vi "Filter Path Node.vi"(7 "Node Path Type":string="To Common Doc Dir", 8 "error in":errorcluster, 11 "Nodes Array in":refnum<k20>[](array[refnum])) -> (0 "error out":errorcluster, 3 "Nodes Array out":refnum<k20>[](array[refnum]))   [LabVIEW 2018, in ".LVLIBP CD XML Updater.lvlib" / "Project XML Editor.lvclass"]
uses:
  Project XML Editor.lvclass
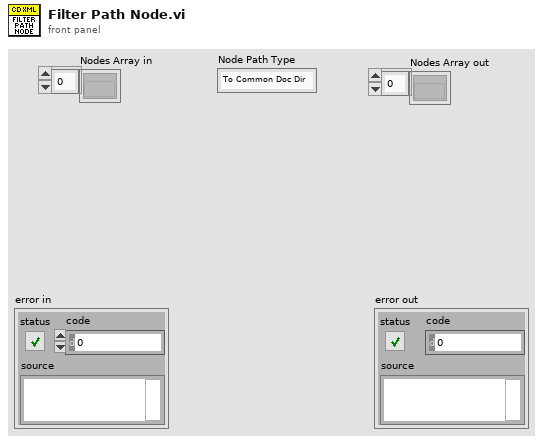
[diagram p1: front panel]
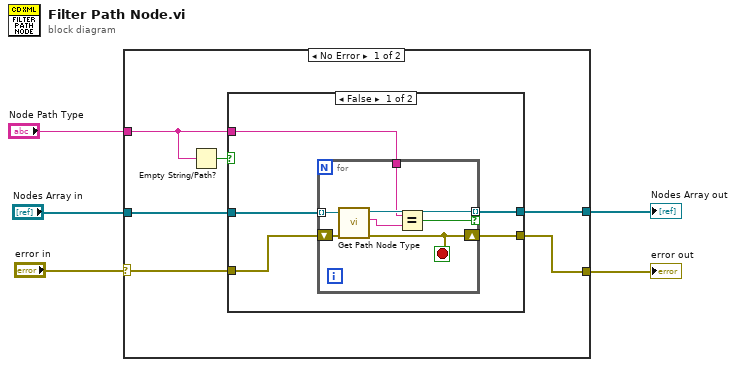
[diagram p0: block diagram]
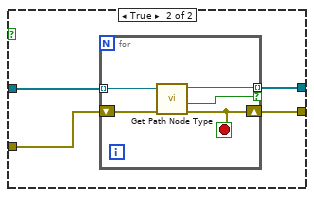
[diagram p2: hidden frame]
diagram:
  n1 = case shown="No Error" "error in" {
    selector: "error in" -> [w8 w33]
    tunnel: "Nodes Array in" -> [w11 w34]
    tunnel: [w10 w34] -> w4
    tunnel: [w9 w33] -> w3
    tunnel: "Node Path Type" -> [w7 _]
    frame No Error {
      n2 = Empty String/Path?(string/path=w7) -> (empty?=w6:bool)
      n3 = case shown="False" w6 {
        tunnel: w11 -> [w16 w27]
        tunnel: [w15 w25] -> w10
        tunnel: [w14 w24] -> w9
        tunnel: w8 -> [w13 w26]
        tunnel: w7 -> [w12 _]
        frame False {
          n4 = for {
            tunnel: [w23] -> w15 mode=indexing if=w22
            tunnel: w16 -> [w21] mode=indexing
            shift-right: [w18] -> w14
            shift-left: w13 -> [w20]
            tunnel: w12 -> [w17]
            stop <- w18 stop-if-true
            n5 = call "Get Path Node Type.vi"("error in (no error)"=w20, "Node ref in"=w21) -> ("error out"=w18:errorcluster, "Path Type out"=w19:string, "Node ref out"=w23:refnum<k20>)  [unwired: 6 in, 1 out]
            n6 = Equal?(x=w17, y=w19) -> (x = y?=w22:bool)
          }
        }
        frame True {
          n7 = for {
            tunnel: [w32] -> w25 mode=indexing if=w28
            tunnel: w27 -> [w31] mode=indexing
            shift-right: [w29] -> w24
            shift-left: w26 -> [w30]
            stop <- w29 stop-if-true
            n8 = call "Get Path Node Type.vi"("error in (no error)"=w30, "Node ref in"=w31) -> ("error out"=w29:errorcluster, "Found ?"=w28:bool, "Node ref out"=w32:refnum<k20>)  [unwired: 6 in, 1 out]
          }
        }
      }
    }
    frame Error {
    }
  }
  "Nodes Array out" <- w4
  "error out" <- w3
